vi "Insight_Laser_Read-Write.vi"(8 "error in (no error)":errorcluster, 9 "String":string, 10 "VISA resource name":refnum<visa-resource-name>, 11 "connection ID":refnum<k5>) -> (0 "error out":errorcluster, 1 "String Out":string, 2 "VISA resource out":refnum<visa-resource-name>, 3 "connection ID out":refnum<k5>, 5 "Numerical Response":dbl)   [LabVIEW 2010]
doc: "Insight Photonic Solutions\n\nThis VI performs read-write operations to-from the Insight Laser. The VI supports either Serial or TCP/IP connections.\n\nver 1.0 - original release"
panel:
  in  "Interface Type":enum16{"Ethernet", "Serial"}(ring)
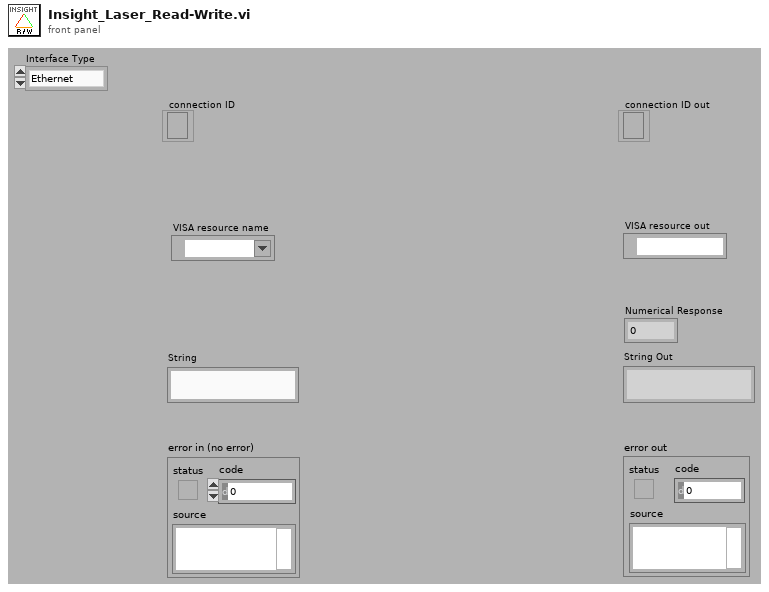
[diagram p1: front panel]
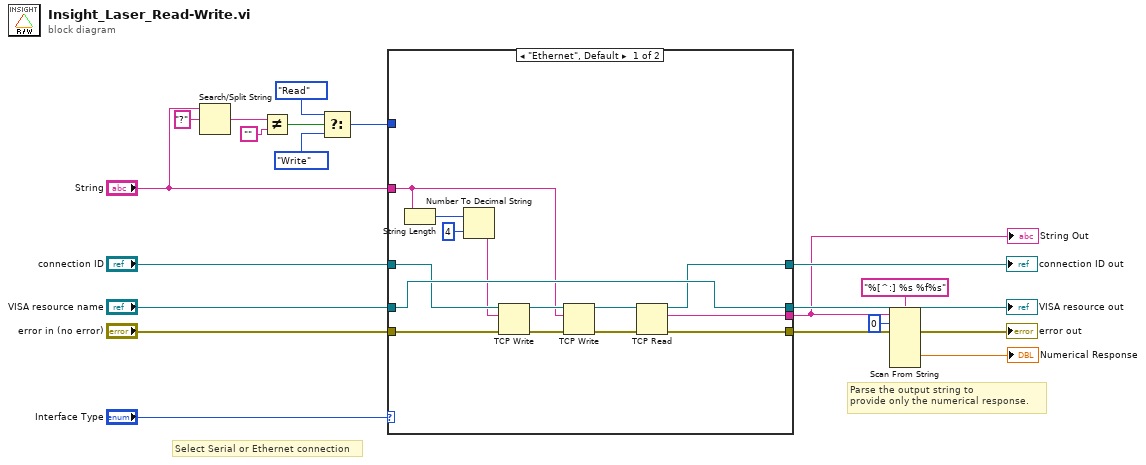
[diagram p0: block diagram]
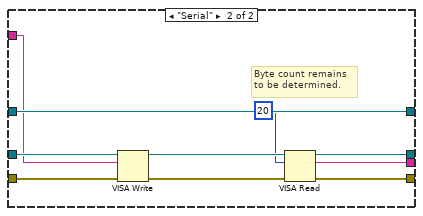
[diagram p2: hidden frame]
diagram:
  # "Parse the output string to\nprovide only the numerical response."
  # "Select Serial or Ethernet connection"
  n1 = Search/Split String(string="String", search string/char (-)="?") -> (match + rest of string=w12:string)  [unwired: 1 in, 2 out]
  n2 = Not Equal?(x=w12, y="") -> (x != y?=w9:bool)
  n3 = Select(t=enum8{"Write", "Read"}."Read" ("Mode"), s=w9, f=enum8{"Write", "Read"}."Write" ("Mode")) -> (s? t:f=w8:enum8{"Write", "Read"})
  n4 = case shown="\"Ethernet\", Default" "Interface Type" {
    tunnel: [w32 w44] -> w5
    tunnel: [w34 w43] -> w20
    tunnel: [w30 w42] -> w3
    tunnel: "VISA resource name" -> [w34 w41]
    tunnel: "error in (no error)" -> [w33 w40]
    tunnel: [w31 w39] -> w17
    tunnel: "connection ID" -> [w29 w39]
    tunnel: "String" -> [w21 w38]
    tunnel: w8 -> [_ _]
    frame "Ethernet", Default {
      n5 = String Length(string=w21) -> (length=w28:i32)
      n6 = Number To Decimal String(number=w28, width (-)=i16 4) -> (decimal integer string=w22:string)
      n7 = TCP Write(connection ID=w29, data in=w22, error in (no error)=w33) -> (connection ID out=w26:refnum<k5>, error out=w25:errorcluster)  [unwired: 1 in, 1 out]
      n8 = TCP Write(connection ID=w26, data in=w21, error in (no error)=w25) -> (connection ID out=w23:refnum<k5>, error out=w24:errorcluster)  [unwired: 1 in, 1 out]
      n9 = TCP Read(connection ID=w23, error in (no error)=w24) -> (connection ID out=w31:refnum<k5>, data out=w30:string, error out=w32:errorcluster)  [unwired: 3 in]
    }
    frame "Serial" {
      # "Byte count remains\nto be determined."
      n10 = VISA Write(VISA resource name=w41, write buffer=w38, error in (no error)=w40) -> (VISA resource name out=w36:refnum<visa-resource-name>, error out=w37:errorcluster)  [unwired: 1 out]
      n11 = VISA Read(VISA resource name=w36, byte count=u32 20, error in (no error)=w37) -> (VISA resource name out=w43:refnum<visa-resource-name>, read buffer=w42:string, error out=w44:errorcluster)  [unwired: 1 out]
    }
  }
  "VISA resource out" <- w20
  "String Out" <- w3
  "connection ID out" <- w17
  n12 = Scan From String(format string="%[^:] %s %f%s", input string=w3, initial scan location=u32 0, error in=w5) -> (error out=→"error out":errorcluster, output 3=→"Numerical Response":dbl)  [unwired: 7 in, 2 out]
